vi "create.vi"(8 "error in (no error)":errorcluster, 9 "Timings":T1, 10 "Settings":T2, 11 "ILCFactory in":refnum<class "ILCFactory.lvclass">) -> (0 "error out":errorcluster, 2 "ILC":refnum<class "ILC.lvclass">, 3 "ILCFactory out":refnum<class "ILCFactory.lvclass">)   [LabVIEW 2016, in "RTILC.lvlib" / "ILCFactory.lvclass"]
uses:
  ILCFactory.lvclass
  DataTypes/ILCSettings.ctl
  ILC/ILC.lvclass
  DataTypes/ILCTimings.ctl
  DataTypes/ILCData.ctl
  DataTypes/ILCConstants.ctl
  DataTypes/ILCCommand.ctl
  DataTypes/ILCScanRates.ctl
  DataTypes/ILCTelemetry.ctl
  DataTypes/ILCResponses.ctl
  Common_RT_Modbus/DataTypes/ExceptionCodes.ctl
  DataTypes/ILCTimestamps.ctl
  ILC/ILC.lvclass/ILC.ctl
  RTILC.lvlib
  Common_RT_Modbus/RTModbus.lvlib
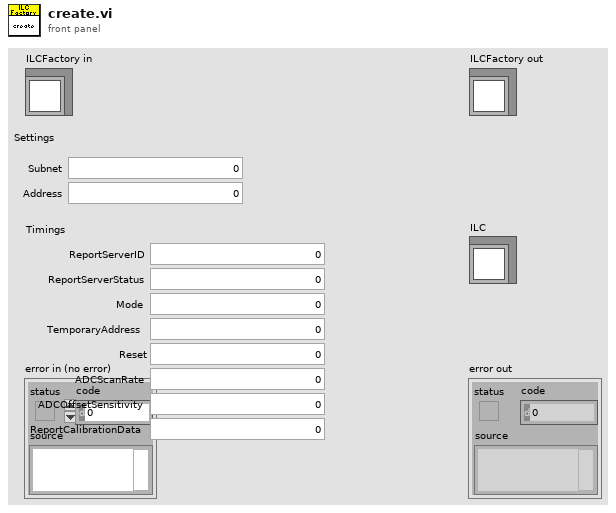
[diagram p1: front panel]
types:
  T1 = typedef "RTILC.lvlib/ILCTimings.ctl" = cluster{"ReportServerID":u32, "ReportServerStatus":u32, "Mode":u32, "TemporaryAddress":u32, "Reset":u32, "ADCScanRate":u32, "ADCOffsetSensitivity":u32, "ReportCalibrationData":u32}
  T2 = typedef "RTILC.lvlib/ILCSettings.ctl" = cluster{"Subnet":u8, "Address":u8}
  T3 = typedef "RTILC.lvlib/ILCData.ctl" = cluster{"Constants":T4, "Command":T5, "Telemetry":T7, "Responses":T8, "Timestamps":T10, "Timings":T1}
  T4 = typedef "RTILC.lvlib/ILCConstants.ctl" = cluster{"Subnet":u8, "Address":u8}
  T5 = typedef "RTILC.lvlib/ILCCommand.ctl" = cluster{"Mode":u16, "TemporaryAddress":u8, "ADCScanRate":T6, "ADCChannel":u8, "ADCOffset":sgl, "ADCSensitivity":sgl}
  T6 = typedef "RTILC.lvlib/ILCScanRates.ctl" = u8
  T7 = typedef "RTILC.lvlib/ILCTelemetry.ctl" = cluster{"UniqueID":u64, "FirmwareType":u8, "NetworkNodeType":u8, "ILCOption":u8, "NetworkNodeOption":u8, "MajorRevision":u8, "MinorRevision":u8, "FirmwareName":string, "Mode":u16, "MajorFault":bool, "MinorFault":bool, "FaultOverride":bool, "MainCalibrationError":bool, "BackupCalibrationError":bool, "UniqueIDCRCMismatch":bool, "AppTypeNodeTypeMismatch":bool, "AppMissing":bool, "AppCRCMismatch":bool, "TEDSNotFound":bool, "TEDS1Mismatch":bool, "TEDS2Mismatch":bool, "WatchdogResetDetected":bool, "BrownoutDetected":bool, "EventTrapResetDetected":bool, "MotorPowerFault":bool, "SSRPowerFault":bool, "AuxPowerFault":bool, "SMCPowerFault":bool, "TemporaryAddress":u8, "ADCScanRate":T6, "MainADCCalibrationK":sgl[], "MainSensorOffset":sgl[], "MainSensorSensitivity":sgl[], "BackupADCCalibrationK":sgl[], "BackupSensorOffset":sgl[], "BackupSensorSensitivity":sgl[]}
  T8 = typedef "RTILC.lvlib/ILCResponses.ctl" = cluster{"ReportServerID":T9, "ReportServerStatus":T9, "Mode":T9, "TemporaryAddress":T9, "Reset":T9, "ADCScanRate":T9, "ADCOffsetSensitivity":T9, "ReportCalibrationData":T9}
  T9 = typedef "RTModbus.lvlib/ExceptionCodes.ctl" = u16
  T10 = typedef "RTILC.lvlib/ILCTimestamps.ctl" = cluster{"ReportServerID":dbl, "ReportServerStatus":dbl, "Mode":dbl, "TemporaryAddress":dbl, "Reset":dbl, "ADCScanRate":dbl, "ADCOffsetSensitivity":dbl, "ReportCalibrationData":dbl}
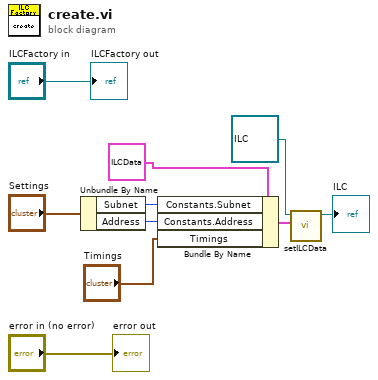
[diagram p0: block diagram]
diagram:
  n1 = Unbundle By Name("Settings") -> ("Subnet"=w8:u8, "Address"=w7:u8)
  n2 = Bundle By Name(cluster=T3 {"Constants"={"Subnet"=0, "Address"=0}, "Command"={"Mode"=0, "TemporaryAddress"=0, "ADCScanRate"=0, "ADCChannel"=0, "ADCOffset"=0.0, "ADCSensitivity"=0.0}, "Telemetry"={"UniqueID"=0, "FirmwareType"=0, "NetworkNodeType"=0, "ILCOption"=0, "NetworkNodeOption"=0, "MajorRevision"=0, "MinorRevision"=0, "FirmwareName"="", "Mode"=0, "MajorFault"=FALSE, "MinorFault"=FALSE, "FaultOverride"=FALSE, "MainCalibrationError"=FALSE, "BackupCalibrationError"=FALSE, "UniqueIDCRCMismatch"=FALSE, "AppTypeNodeTypeMismatch"=FALSE, "AppMissing"=FALSE, "AppCRCMismatch"=FALSE, "TEDSNotFound"=FALSE, "TEDS1Mismatch"=FALSE, "TEDS2Mismatch"=FALSE, "WatchdogResetDetected"=FALSE, "BrownoutDetected"=FALSE, "EventTrapResetDetected"=FALSE, "MotorPowerFault"=FALSE, "SSRPowerFault"=FALSE, "AuxPowerFault"=FALSE, "SMCPowerFault"=FALSE, "TemporaryAddress"=0, "ADCScanRate"=0, "MainADCCalibrationK"=[], "MainSensorOffset"=[], "MainSensorSensitivity"=[], "BackupADCCalibrationK"=[], "BackupSensorOffset"=[], "BackupSensorSensitivity"=[]}, "Responses"={"ReportServerID"=0, "ReportServerStatus"=0, "Mode"=0, "TemporaryAddress"=0, "Reset"=0, "ADCScanRate"=0, "ADCOffsetSensitivity"=0, "ReportCalibrationData"=0}, "Timestamps"={"ReportServerID"=0.0, "ReportServerStatus"=0.0, "Mode"=0.0, "TemporaryAddress"=0.0, "Reset"=0.0, "ADCScanRate"=0.0, "ADCOffsetSensitivity"=0.0, "ReportCalibrationData"=0.0}, "Timings"={"ReportServerID"=0, "ReportServerStatus"=0, "Mode"=0, "TemporaryAddress"=0, "Reset"=0, "ADCScanRate"=0, "ADCOffsetSensitivity"=0, "ReportCalibrationData"=0}} ("ILCData"), "Constants.Subnet"=w8, "Constants.Address"=w7, "Timings"="Timings") -> (w5:T3)
  n3 = call "setILCData.vi"("ILCData"=w5, "ILC in"=refnum<class "ILC.lvclass"> refnum ("RTILC.lvlib:ILC.lvclass")) -> ("ILC out"=→"ILC":refnum<class "ILC.lvclass">)  [unwired: 9 in]
  "error out" <- "error in (no error)"
  "ILCFactory out" <- "ILCFactory in"
